vi "Default_Initialize_IMU.vi"(8 "error in (no error)":errorcluster) -> (0 "error out":errorcluster, 2 "Gyro FSR":i32, 3 "data out":T1)   [LabVIEW 2014]
uses:
  <userlib>/test_IMU/test_IMU.lvlib
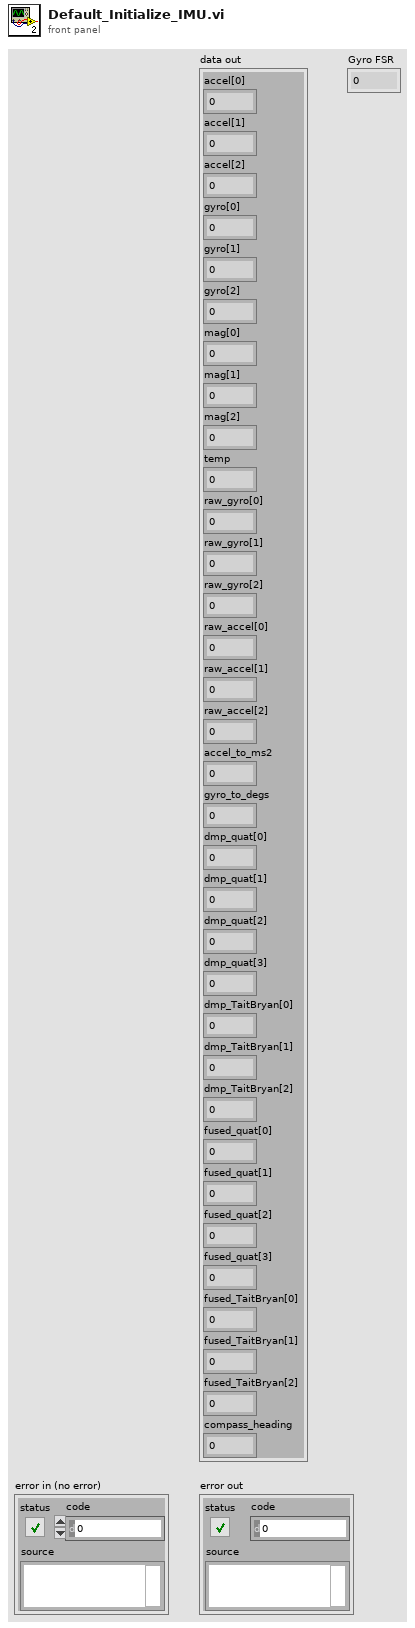
[diagram p1: front panel]
types:
  T1 = cluster{"accel[0]":sgl, "accel[1]":sgl, "accel[2]":sgl, "gyro[0]":sgl, "gyro[1]":sgl, "gyro[2]":sgl, "mag[0]":sgl, "mag[1]":sgl, "mag[2]":sgl, "temp":sgl, "raw_gyro[0]":i16, "raw_gyro[1]":i16, "raw_gyro[2]":i16, "raw_accel[0]":i16, "raw_accel[1]":i16, "raw_accel[2]":i16, "accel_to_ms2":sgl, "gyro_to_degs":sgl, "dmp_quat[0]":sgl, "dmp_quat[1]":sgl, "dmp_quat[2]":sgl, "dmp_quat[3]":sgl, "dmp_TaitBryan[0]":sgl, "dmp_TaitBryan[1]":sgl, "dmp_TaitBryan[2]":sgl, "fused_quat[0]":sgl, "fused_quat[1]":sgl, "fused_quat[2]":sgl, "fused_quat[3]":sgl, "fused_TaitBryan[0]":sgl, "fused_TaitBryan[1]":sgl, "fused_TaitBryan[2]":sgl, "compass_heading":sgl}
  T2 = cluster{"accel_fsr":u32, "gyro_fsr":u32, "gyro_dlpf":u32, "accel_dlpf":u32, "enable_magnetometer":i32, "dmp_sample_rate":i32, "orientation":u32, "compass_mix_factor":i32, "dmp_interrupt_priority":i32, "show_warnings":i32}
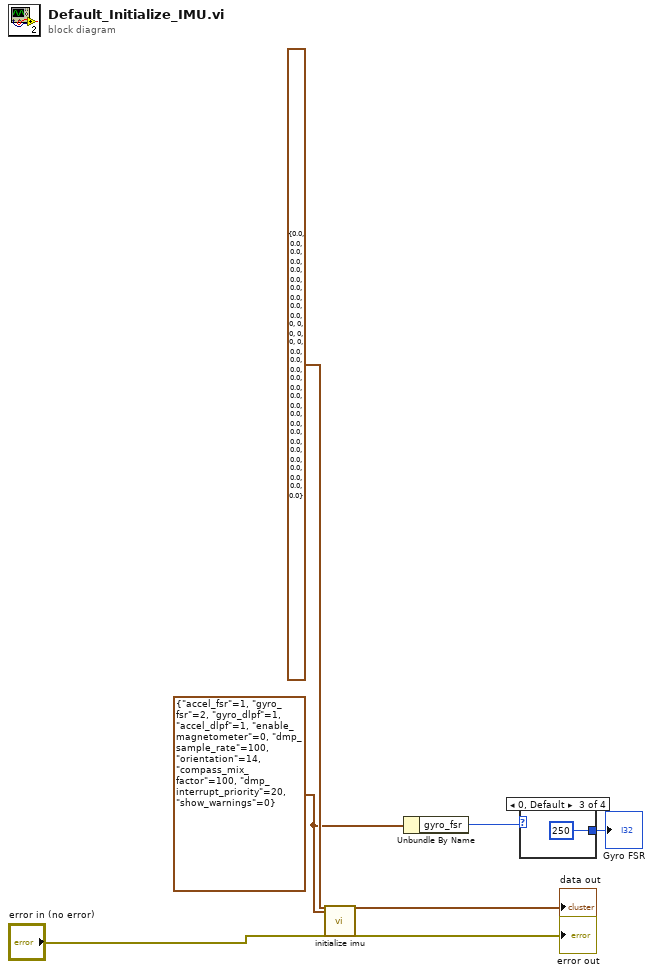
[diagram p0: block diagram]
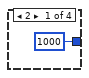
[diagram p2: hidden frame]
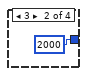
[diagram p3: hidden frame]
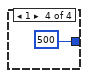
[diagram p4: hidden frame]
diagram:
  w3 = T2 {"accel_fsr"=1, "gyro_fsr"=2, "gyro_dlpf"=1, "accel_dlpf"=1, "enable_magnetometer"=0, "dmp_sample_rate"=100, "orientation"=14, "compass_mix_factor"=100, "dmp_interrupt_priority"=20, "show_warnings"=0} ("conf")
  n1 = call <userlib>:"initialize imu.vi"("data"=T1 {"accel[0]"=0.0, "accel[1]"=0.0, "accel[2]"=0.0, "gyro[0]"=0.0, "gyro[1]"=0.0, "gyro[2]"=0.0, "mag[0]"=0.0, "mag[1]"=0.0, "mag[2]"=0.0, "temp"=0.0, "raw_gyro[0]"=0, "raw_gyro[1]"=0, "raw_gyro[2]"=0, "raw_accel[0]"=0, "raw_accel[1]"=0, "raw_accel[2]"=0, "accel_to_ms2"=0.0, "gyro_to_degs"=0.0, "dmp_quat[0]"=0.0, "dmp_quat[1]"=0.0, "dmp_quat[2]"=0.0, "dmp_quat[3]"=0.0, "dmp_TaitBryan[0]"=0.0, "dmp_TaitBryan[1]"=0.0, "dmp_TaitBryan[2]"=0.0, "fused_quat[0]"=0.0, "fused_quat[1]"=0.0, "fused_quat[2]"=0.0, "fused_quat[3]"=0.0, "fused_TaitBryan[0]"=0.0, "fused_TaitBryan[1]"=0.0, "fused_TaitBryan[2]"=0.0, "compass_heading"=0.0}, "IMU_Config_t"=w3, "error in (no error)"="error in (no error)") -> ("data out"=→"data out":T1, "error out"=→"error out":errorcluster)  [unwired: 22 in, 1 out]
  n2 = Unbundle By Name(w3) -> ("gyro_fsr"=w2:u32)
  n3 = case shown="0, Default" w2 {
    tunnel: [1000 2000 250 500] -> w1
    frame 2 {
    }
    frame 3 {
    }
    frame 0, Default {
    }
    frame 1 {
    }
  }
  "Gyro FSR" <- w1
